vi "Initialize.vi"(8 "error in (no error)":errorcluster caption="错误输入（无错误）", 11 "Section输入":refnum<class "Section.lvclass">) -> (0 "error out":errorcluster caption="错误输出", 3 "Section输出":refnum<class "Section.lvclass">)   [LabVIEW 2013, in "Hierarchy Framework.lvlib" / "Section.lvclass"]
uses:
  Section.lvclass
  Item/Item.lvclass
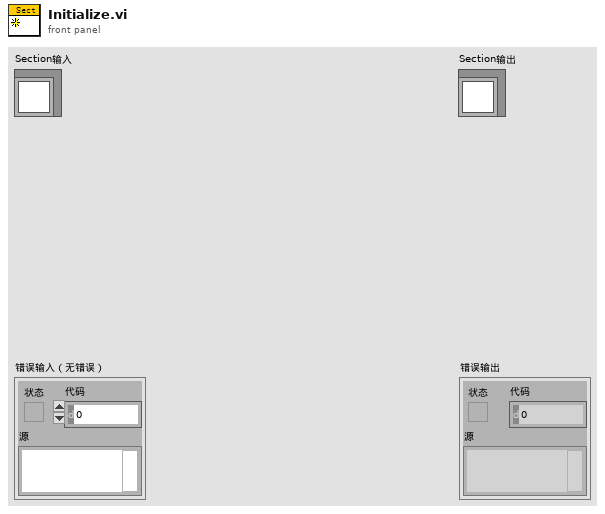
[diagram p1: front panel]
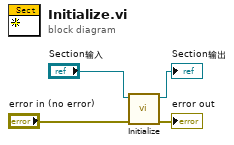
[diagram p0: block diagram]
diagram:
  n1 = call-parent "Initialize.vi"("error in (no error)"="error in (no error)", "Item输入"="Section输入") -> ("error out"=→"error out":errorcluster, "Item输出"=→"Section输出":refnum<class "Section.lvclass">)  [unwired: 8 in]
